vi "Page_Service_Config_ReadAll.vi"(6 "ctl references":T1, 8 "error in (no error)":errorcluster, 11 "AB_RESTfulWebService in":refnum<class "AB_RESTfulWebService.lvclass">) -> (0 "error out":errorcluster, 3 "AB_RESTfulWebService out":refnum<class "AB_RESTfulWebService.lvclass">)   [LabVIEW 2020, in "AB_RESTfulWebService.lvclass"]
uses:
  <vilib>/AppBuilder/AB_Classes/RESTful/AB_RESTfulWebService.lvclass
  <resource>/Framework/Providers/Builds/AppBuilder/AB_UI_Page_Service_Config_References.ctl
  <vilib>/AppBuilder/AB_Classes/RESTful/AB_RESTfulWebService.lvclass/AB_RESTfulWebService.ctl
  <vilib>/AppBuilder/AB_Classes/WebService/AB_WebService.lvclass
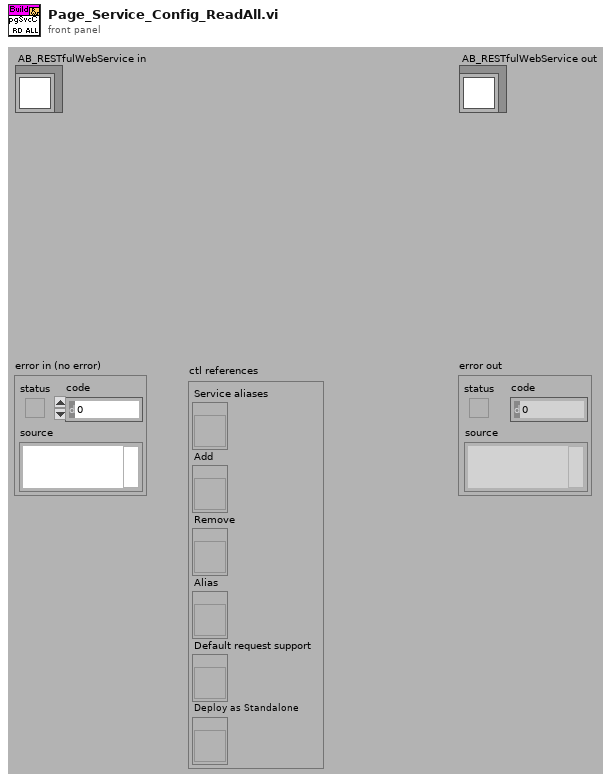
[diagram p1: front panel]
types:
  T1 = typedef "AB_UI_Page_Service_Config_References.ctl" = cluster{"Service aliases":refnum<vi>, "Add":refnum<vi>, "Remove":refnum<vi>, "Alias":refnum<vi>, "Default request support":refnum<vi>, "Deploy as Standalone":refnum<vi>}
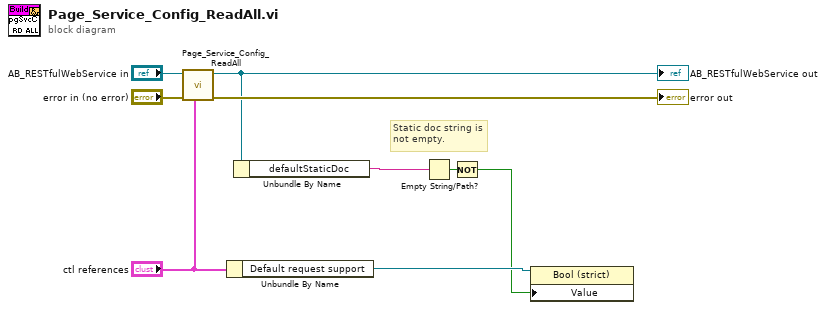
[diagram p0: block diagram]
diagram:
  # "Static doc string is  not empty."
  n1 = call-parent "Page_Service_Config_ReadAll.vi"("ctl references"="ctl references", "error in (no error)"="error in (no error)", "AB_WebService in"="AB_RESTfulWebService in") -> ("error out"=→"error out":errorcluster, "AB_WebService out"=w6:refnum<class "AB_RESTfulWebService.lvclass">)  [unwired: 7 out]
  "AB_RESTfulWebService out" <- w6
  n2 = Unbundle By Name("ctl references") -> ("Default request support"=w3:refnum<vi>)
  n3 = Unbundle By Name(w6) -> ("defaultStaticDoc"=w4:string)
  n4 = Empty String/Path?(string/path=w4) -> (empty?=w2:bool)
  n5 = Not(x=w2) -> (.not. x?=w1:bool)
  n6 = property class="Bool (strict)"(reference=w3, "Value"=w1) -> ()  [unwired: 1 in, 2 out]
